vi "Daniel Kraus.vi"() -> ()   [LabVIEW 2010]
uses:
  <vilib>/addons/database/Auxilliary.llb/DB Tools Cursor Type.ctl
  <vilib>/addons/database/NI_Database_API.lvlib
  <vilib>/addons/database/Connection.llb/DB Tools Open Connec (Path).vi
  <vilib>/addons/database/Recordset.llb/Rec Fetch Recordset Data (R).vi
  <vilib>/addons/database/Connection.llb/Conn Execute.vi
  <vilib>/addons/database/_DB Variant To Data/Database Variant To Data.xnode
  <vilib>/addons/database/Recordset.llb/Rec Destroy - Connection.vi
panel:
  in  "Create\nTable?":bool=TRUE
  in  "Table Name":string="Danial"
  out "recordset data":variant[][](array[variant])
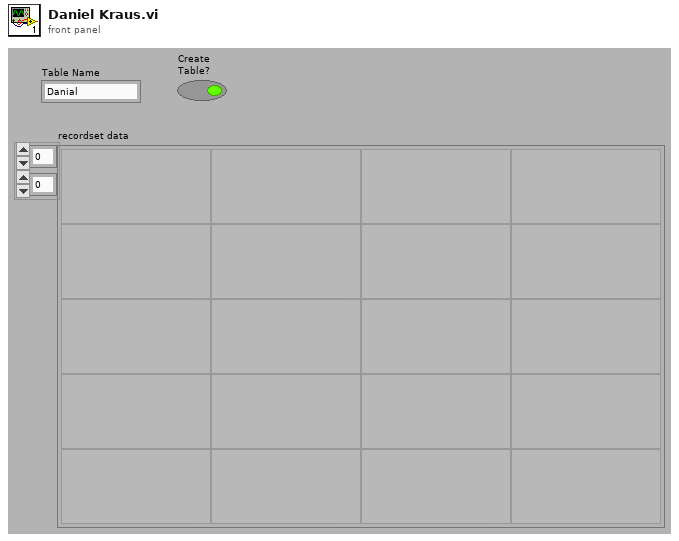
[diagram p1: front panel]
types:
  T1 = typedef "NI_Database_API.lvlib/DB Tools Cursor Type.ctl" = enum16{"forward-only", "keyset", "dynamic", "static"}
  T2 = typedef "NI_Database_API.lvlib/Conn ObjectReference.ctl" = refnum<k1>
  T3 = typedef "NI_Database_API.lvlib/Rec ObjectReference.ctl" = refnum<k1>
  T4 = cluster{"data":i32, "data":string, "data":string, "data":string}
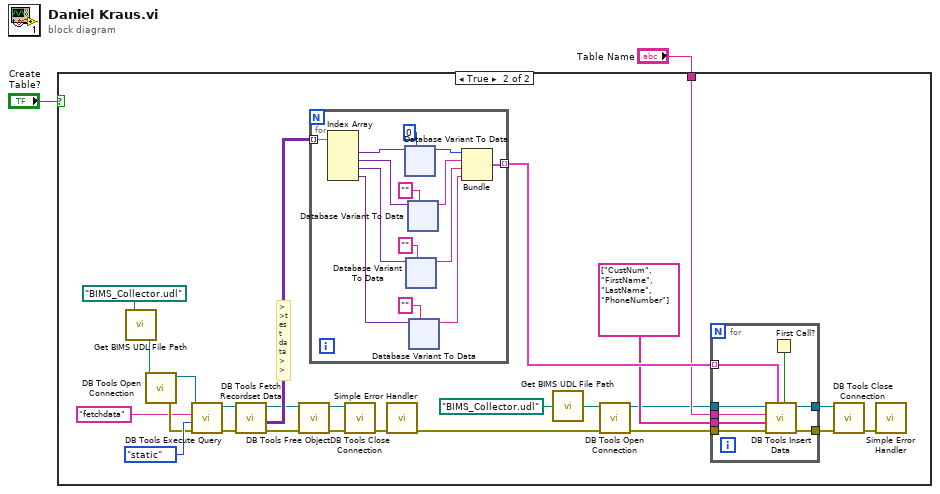
[diagram p0: block diagram]
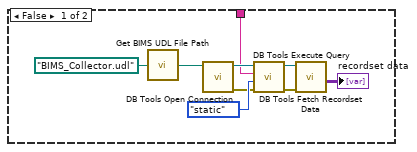
[diagram p2: hidden frame]
diagram:
  n1 = case shown="True" "Create\nTable?" {
    tunnel: "Table Name" -> [w4 w20]
    frame False {
      n2 = call "Get BIMS UDL File Path.vi"("UDL file name"=path "BIMS_Collector.udl") -> ("Full UDL file path"=w8:path)
      n3 = call-poly <vilib>:"DB Tools Open Connection.vi"("connection information"=w8) -> ("error out"=w7:errorcluster, "connection reference"=w6:T2)  [unwired: 4 in, 3 out]
      n4 = call-poly <vilib>:"DB Tools Execute Query.vi"("error in (no error)"=w7, "cursor type"=DB_Tools_Cursor_Type."static", "SQL query"=w4, "connection reference"=w6) -> ("error out"=w9:errorcluster, "recordset reference"=w5:T3)  [unwired: 4 out]
      n5 = call-poly <vilib>:"DB Tools Fetch Recordset Data.vi"("error in (no error)"=w9, "recordset reference"=w5) -> ("recordset data"=→"recordset data":variant[][])  [unwired: 5 out]
    }
    frame True {
      # ">>test data>>"
      n6 = call "Get BIMS UDL File Path.vi"("UDL file name"=path "BIMS_Collector.udl") -> ("Full UDL file path"=w31:path)
      n7 = call-poly <vilib>:"DB Tools Open Connection.vi"("connection information"=w31) -> ("error out"=w30:errorcluster, "connection reference"=w23:T2)  [unwired: 4 in, 3 out]
      n8 = call-poly <vilib>:"DB Tools Execute Query.vi"("error in (no error)"=w30, "cursor type"=DB_Tools_Cursor_Type."static", "SQL query"="fetchdata", "connection reference"=w23) -> ("error out"=w32:errorcluster, "recordset reference"=w29:T3)  [unwired: 4 out]
      n9 = call-poly <vilib>:"DB Tools Fetch Recordset Data.vi"("error in (no error)"=w32, "recordset reference"=w29) -> ("error out"=w24:errorcluster, "recordset data"=w27:variant[][], "recordset reference out"=w25:T3)  [unwired: 3 out]
      n10 = call-poly <vilib>:"DB Tools Free Object.vi"("error in (no error)"=w24, "recordset reference"=w25) -> ("error out"=w17:errorcluster, "connection reference"=w18:T2)  [unwired: 8 out]
      n11 = for {
        tunnel: [w58] -> w26 mode=indexing
        tunnel: w27 -> [w57] mode=indexing
        n12 = Index Array(array=w57) -> (element #1=w56:variant, element #2=w53:variant, element #3=w46:variant, element #4=w45:variant)  [unwired: 4 in]
        n13 = xnode ("Database Variant To Data")("database variant"=w56, "type"=0) -> ("data"=w55:i32)  [unwired: 1 in, 1 out]
        n14 = xnode "Database Variant To Data"("database variant"=w46, "type"="") -> ("data"=w49:string)  [unwired: 1 in, 1 out]
        n15 = xnode "Database Variant To Data"("database variant"=w53, "type"="") -> ("data"=w51:string)  [unwired: 1 in, 1 out]
        n16 = xnode "Database Variant To Data"("database variant"=w45, "type"="") -> ("data"=w47:string)  [unwired: 1 in, 1 out]
        n17 = Bundle("data"=w55, "data"=w51, "data"=w49, "data"=w47) -> (w58:T4)  [unwired: 1 out]
      }
      n18 = call <vilib>:"DB Tools Close Connection.vi"("error in (no error)"=w17, "connection reference"=w18) -> ("error out"=w19:errorcluster)  [unwired: 5 out]
      n19 = call <vilib>:"Simple Error Handler.vi"("error in (no error)"=w19) -> ("error out"=w12:errorcluster)  [unwired: 1 in, 7 out]
      n20 = call "Get BIMS UDL File Path.vi"("UDL file name"=path "BIMS_Collector.udl") -> ("Full UDL file path"=w16:path)
      n21 = call-poly <vilib>:"DB Tools Open Connection.vi"("error in (no error)"=w12, "connection information"=w16) -> ("error out"=w13:errorcluster, "connection reference"=w14:T2)  [unwired: 3 in, 3 out]
      n22 = for {
        tunnel: [w44] -> w36
        tunnel: [w43] -> w35
        tunnel: w14 -> [w42]
        tunnel: w13 -> [w41]
        tunnel: w20 -> [w40]
        tunnel: w26 -> [w38] mode=indexing
        tunnel: string[] ["CustNum", "FirstName", "LastName", "PhoneNumber"] ("columns") -> [w37]
        n23 = First Call?() -> (First Call?: T/F=w39:bool)
        n24 = call <vilib>:"DB Tools Insert Data.vi"("create table? (F)"=w39, "data"=w38, "error in (no error)"=w41, "columns"=w37, "table"=w40, "connection reference"=w42) -> ("error out"=w43:errorcluster, "connection reference out"=w44:T2)  [unwired: 1 in, 3 out]
      }
      n25 = call <vilib>:"DB Tools Close Connection.vi"("error in (no error)"=w35, "connection reference"=w36) -> ("error out"=w34:errorcluster)  [unwired: 5 out]
      n26 = call <vilib>:"Simple Error Handler.vi"("error in (no error)"=w34) -> ()  [unwired: 1 in, 8 out]
    }
  }
